vi "Actor Core.vi"(8 "error in":errorcluster, 11 "Nested in":refnum<class "TCP 380.lvclass">) -> (0 "error out":errorcluster, 3 "Actor out":refnum<class "Actor.lvclass">)   [LabVIEW 2021, in "TCP 380.lvclass"]
doc: "(<B>Filename</B>: Actor Framework.lvlib:Actor.lvclass:Actor Core.vi)\n\nReceives messages to the actor, reacts to them, and initiates any error handling that may shut the actor down.\n\nDescendant classes may override this VI to append parallel tasks for the actor to complete while it handles messages. Overrides use the Call Parent Method node."
uses:
  TCP 380.lvclass
  <vilib>/ActorFramework/Actor/Actor.lvclass
  C:/Program Files/National Instruments/LabVIEW 2021/vi.lib/ActorFramework/Actor/Actor.lvclass
  TCP 380.lvclass/TCP 380.ctl
  <vilib>/ActorFramework/Actor/Actor.lvclass/Actor.ctl
  <vilib>/ActorFramework/Message Enqueuer/Message Enqueuer.lvclass/Message Enqueuer.ctl
  Vacuum Pumps/Vacuum Pumps Messages/Toggle Power Msg/Toggle Power Msg.lvclass/Toggle Power Msg.ctl
  <vilib>/ActorFramework/Message Enqueuer/Init from Existing Queue.vi
  <vilib>/ActorFramework/Message Enqueuer/Enqueue.vi
  <vilib>/ActorFramework/Stop Msg/Stop Msg.lvclass
  C:/Program Files/National Instruments/LabVIEW 2021/vi.lib/ActorFramework/Message/Message.lvclass
  Vacuum Pumps/Vacuum Pumps Messages/Toggle Power Msg/Toggle Power Msg.lvclass
  <vilib>/ActorFramework/Message Priority Queue/Priority Enqueue.vi
  <vilib>/ActorFramework/Message Enqueuer/Message Enqueuer.lvclass
  <vilib>/MGI/Panel Manager/Panel Actor/Panel Actor/Panel Actor.lvclass
panel:
  in  "Upd State":bool
  out "K2":bool caption="Error"
  out "K1":bool caption="Nominal"
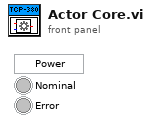
[diagram p1: front panel]
types:
  T1 = cluster{"Stop":refnum<user-event>, "K2":refnum<user-event>, "K1":refnum<user-event>}
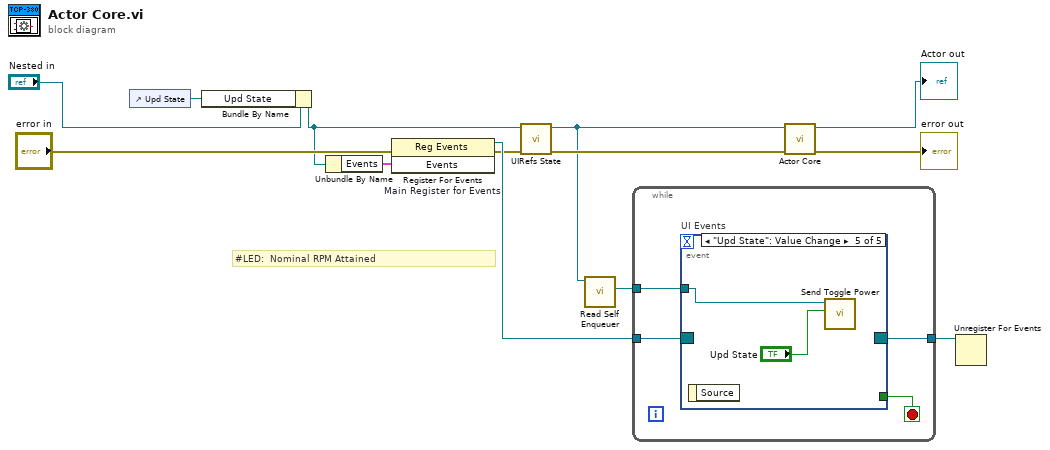
[diagram p0: block diagram]
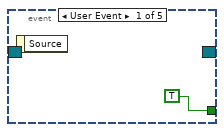
[diagram p2: hidden frame]
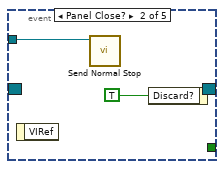
[diagram p3: hidden frame]
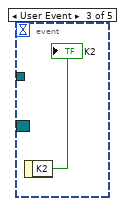
[diagram p4: hidden frame]
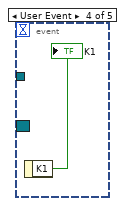
[diagram p5: hidden frame]
diagram:
  # "#LED:  Nominal RPM Attained"
  n1 = control-ref of="Upd State"() -> (w2:refnum<vi>)
  n2 = Bundle By Name(cluster="Nested in", "Upd State"=w2) -> (w3:refnum<class "TCP 380.lvclass">)
  n3 = Unbundle By Name(w3) -> ("Events"=w10:T1)
  n4 = register-events "Main Register for Events"(error in="error in", w10) -> (reference out=w11:refnum<event-registration>, error out=w6:errorcluster)  [unwired: 1 in]
  n5 = call "UIRefs State.vi"("error in (no error)"=w6, "TCP 380 in"=w3) -> ("error out"=w5:errorcluster, "TCP 380 out"=w4:refnum<class "TCP 380.lvclass">)  [unwired: 8 in]
  n6 = call <vilib>:"Read Self Enqueuer.vi"("Actor"=w4) -> ("Self Enqueuer"=w8:refnum<class "Message Enqueuer.lvclass">)  [unwired: 10 in]
  n7 = while {
    tunnel: w11 -> [w17]
    tunnel: [w15] -> w9
    tunnel: w8 -> [w14]
    stop <- w16 stop-if-true
    n8 = event "UI Events" shown="[4] \"Upd State\": Value Change" {
      selector: w17 -> [_ _ _ _ _]
      dyn-events: [_ _ _ _ _] -> w15
      timeout: _ -> [_ _ _ _ _]
      tunnel: [TRUE _ _ _ _] -> w16
      tunnel: w14 -> [_ w19 _ _ w24]
      event User Event {
        n9 = event-data() -> ()  [unwired: 1 in, 1 out]
      }
      event Panel Close? {
        n10 = event-data() -> ()  [unwired: 1 in, 1 out]
        n11 = call <vilib>:"Send Normal Stop.vi"("Message Enqueuer"=w19) -> ()  [unwired: 10 in, 1 out]
        n12 = event-data("Discard?"=TRUE) -> ()  [unwired: 1 in, 1 out]
      }
      event User Event {
        n13 = event-data() -> ("K2"=→"K2":bool)  [unwired: 1 in]
      }
      event User Event {
        n14 = event-data() -> ("K1"=→"K1":bool)  [unwired: 1 in]
      }
      event "Upd State": Value Change {
        n15 = event-data() -> ()  [unwired: 1 in, 1 out]
        n16 = call "Send Toggle Power.vi"("Power On?"="Upd State", "Message Enqueuer"=w24) -> ()  [unwired: 8 in, 2 out]
      }
    }
  }
  n17 = call-parent "Actor Core.vi"("error in"=w5, "Panel Actor in"=w4) -> ("error out"=→"error out":errorcluster, "Actor out"=→"Actor out":refnum<class "Actor.lvclass">)  [unwired: 8 in]
  n18 = Unregister For Events(event registration refnum=w9) -> ()  [unwired: 1 in, 1 out]
